vi "Update UI.vi"(11 "Instr in":refnum<class "Instr Actor.lvclass">) -> ()   [LabVIEW 2014, in "Instrument Library.lvlib" / "Instr Actor.lvclass"]
uses:
  Instr Actor.lvclass
  Instr Actor.lvclass/Instr Actor.ctl
  reusable/Command/Command.lvclass
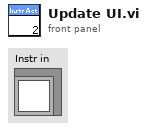
[diagram p1: front panel]
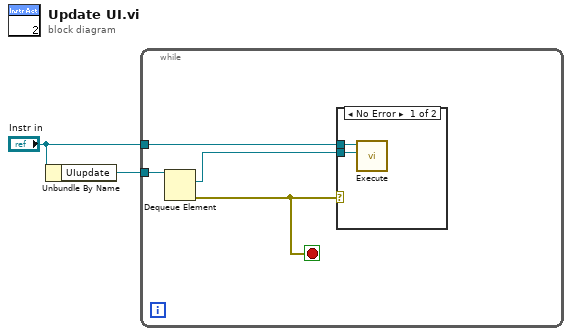
[diagram p0: block diagram]
diagram:
  n1 = Unbundle By Name("Instr in") -> ("UIupdate"=w2:refnum<queue>)
  n2 = while {
    tunnel: w2 -> [w6]
    tunnel: "Instr in" -> [w5]
    stop <- w3 stop-if-true
    n3 = Dequeue Element(queue=w6) -> (element=w4:refnum<class "Command.lvclass">, error out=w3:errorcluster)  [unwired: 2 in, 2 out]
    n4 = case shown="No Error" w3 {
      tunnel: w5 -> [w8 _]
      tunnel: w4 -> [w7 _]
      frame No Error {
        n5 = call-dynamic "Execute.vi"("Command in"=w7, "Object In"=w8) -> ()  [unwired: 8 in, 2 out]
      }
      frame Error {
      }
    }
  }
